vi "Property is Enum.vi"(0 "SLSC Remote in":refnum<class "SLSC Remote.lvclass">, 5 "property":refnum<k21>, 11 "error in (no error)":errorcluster) -> (4 "SLSC Remote out":refnum<class "SLSC Remote.lvclass">, 6 "property out":refnum<k21>, 10 "Prop.IsEnum":bool, 15 "error out":errorcluster)   [LabVIEW 2015, in "SLSC Remote.lvclass"]
uses:
  SLSC Remote.lvclass
  <vilib>/NI/i3 JSON/JSON Generation/Create Value Files/Create Value - Object.vi
  <vilib>/NI/i3 JSON/JSON Generation/Add Object Parameter Files/Add Object Parameter - String.vi
  <vilib>/NI/NI JSONRPC Server Framework/Classes/Server/Format Client Request (Auto-Increment).vi
  <vilib>/httpClient/POSTBuffer.vi
  <vilib>/NI/i3 JSON/JSON Parsing/Get Object Parameter Files/Get Object Parameter - Boolean.vi
  <vilib>/NI/NI JSONRPC Server Framework/Classes/Server/JSONRPC Server.lvclass
  <vilib>/NI/i3 JSON/i3-json.lvlib
  <vilib>/httpClient/LabVIEWHTTPClient.lvlib
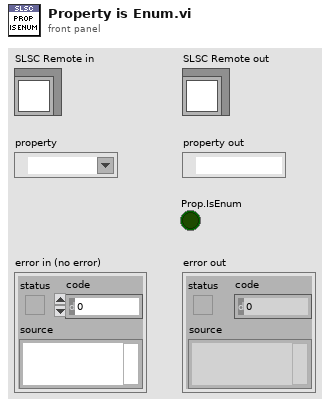
[diagram p1: front panel]
types:
  T1 = typedef "LabVIEWHTTPClient.lvlib/ClientHandle.ctl" = refnum<k1>
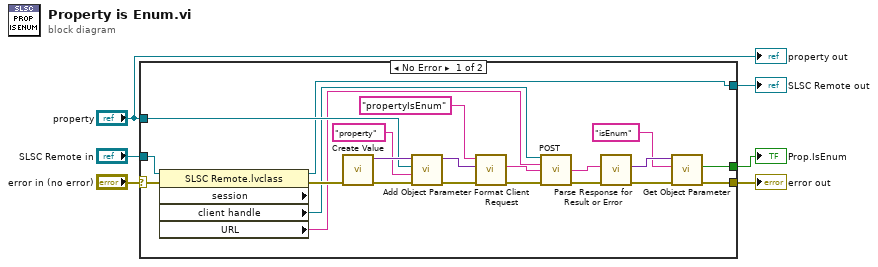
[diagram p0: block diagram]
diagram:
  n1 = case shown="No Error" "error in (no error)" {
    selector: "error in (no error)" -> [w23 w29]
    tunnel: "property" -> [w27 _]
    tunnel: "SLSC Remote in" -> [w25 w30]
    tunnel: [w24 w30] -> w3
    tunnel: [w10 w29] -> w4
    tunnel: [w7 _] -> w2
    frame No Error {
      n2 = property class="SLSC Remote.lvclass" props=["session", "client handle", "URL"](reference=w25, error in=w23) -> (reference out=w24:refnum<class "SLSC Remote.lvclass">, error out=w22:errorcluster, "client handle"=w16:T1, "URL"=w15:string)  [unwired: 1 out]
      n3 = call-poly <vilib>:"Create Value.vi"("error in (no error)"=w22) -> ("error out"=w21:errorcluster, "JSON Tree"=w28:variant)  [unwired: 9 in]
      n4 = call-poly <vilib>:"Add Object Parameter.vi"("error in (no error)"=w21, "Name"="property", "String"=w27, "JSON Tree in (JSON Object)"=w28) -> ("error out"=w20:errorcluster, "JSON Tree out (JSON Object)"=w17:variant)  [unwired: 6 in]
      n5 = call-poly <vilib>:"Format Client Request.vi"("error in (no error)"=w20, "params"=w17, "method"="propertyIsEnum") -> ("error out"=w14:errorcluster, "Request String"=w18:string)  [unwired: 7 in]
      n6 = call-poly <vilib>:"POST.vi"("client handle"=w16, "url"=w15, "buffer"=w18, "error in (no error)"=w14) -> ("body"=w13:string, "error out"=w12:errorcluster)  [unwired: 8 in, 2 out]
      n7 = call <vilib>:"Parse Response for Result or Error.vi"("error in"=w12, "Response String In"=w13) -> ("error out"=w11:errorcluster, "Result or Error Data"=w9:variant)  [unwired: 8 in]
      n8 = call-poly <vilib>:"Get Object Parameter.vi"("error in (no error)"=w11, "Parameter Name"="isEnum", "JSON Tree In (JSON Object)"=w9) -> ("error out"=w10:errorcluster, "Boolean Value"=w7:bool)  [unwired: 5 in, 2 out]
    }
    frame Error {
    }
  }
  "error out" <- w4
  "SLSC Remote out" <- w3
  "Prop.IsEnum" <- w2
  "property out" <- "property"
